vi "GetRtModeStr.vi"(8 "错误输入（无错误）":errorcluster, 9 "收发模式索引":u8, 10 "字符串分配空间大小":u32, 11 "收发方式描述":string) -> (0 "错误输出":errorcluster, 3 "收发方式描述":string)   [LabVIEW 2014]
uses:
  X86Dll/ZXUTConfigMgr.dll
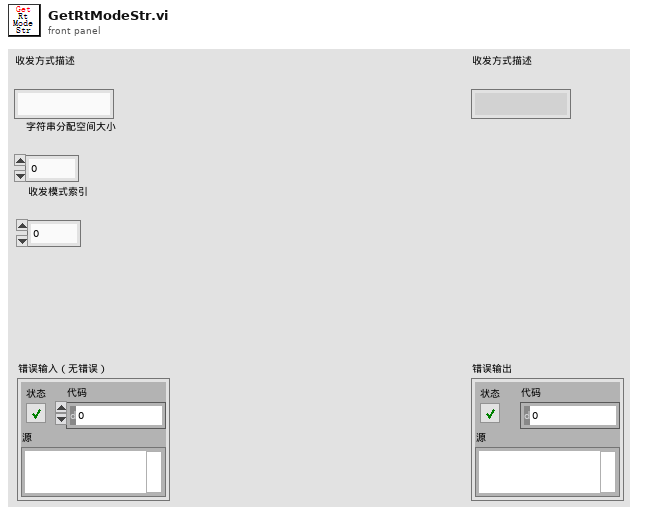
[diagram p1: front panel]
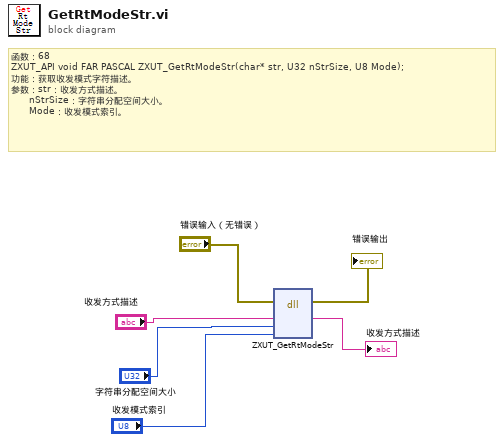
[diagram p0: block diagram]
diagram:
  # "函数：68\nZXUT_API void\tFAR PASCAL ZXUT_GetRtModeStr(char* str, U32 nStrSize, U8 Mode);\n功能：获取收发模式字符描述。\n参数：str：收发方式描述。\n      nStrSize：字符串分配空间大小。\n      Mode：收发模式索引。"
  n1 = dll-call lib="D:/Software/Utrasonic on-line monitoring/X86Dll/ZXUTConfigMgr.dll" fn="ZXUT_GetRtModeStr"(error in="错误输入（无错误）", "str"="收发方式描述", "nStrSize"="字符串分配空间大小", "Mode"="收发模式索引") -> (error out=→"错误输出":errorcluster, "str"=→"收发方式描述":string)  [unwired: 5 in, 1 out]
